vi "custom_func_xt.vi"(7 "func":string="x^2 " caption="y = f(x)", 8 "error in (no error)":errorcluster, 9 "N":i32=10, 10 "dx":dbl=1.0 format="%#_13g", 11 "x0":dbl=1.0 format="%#_13g") -> (0 "error out":errorcluster, 2 "y_vals":dbl[](array[numeric])=[1.0, 4.0, 9.0, 16.0, 25.0, 36.0, 49.0, 64.0, 81.0, 100.0])   [LabVIEW 2017, in "tools.lvlib"]
uses:
  tools.lvlib
  <vilib>/gmath/NI_Gmath.lvlib
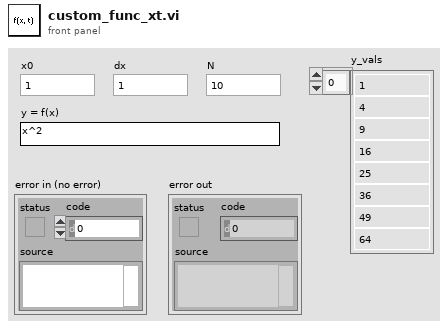
[diagram p1: front panel]
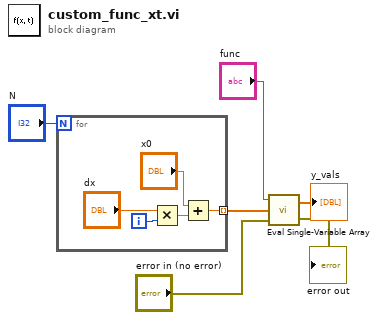
[diagram p0: block diagram]
diagram:
  n1 = for {
    N: "N" -> [_]
    tunnel: [w7] -> w3 mode=indexing
    i -> [w11]
    n2 = Multiply(x="dx", y=w11) -> (x*y=w9:dbl)
    n3 = Add(x="x0", y=w9) -> (x+y=w7:dbl)
  }
  n4 = call <vilib>:"Eval Single-Variable Array.vi"("error in (no error)"="error in (no error)", "X Values"=w3, "formula"="func") -> ("error out"=→"error out":errorcluster, "Y Values"=→"y_vals":dbl[])
